vi "WRO_Main.vi"() -> ()   [LabVIEW 2014]
uses:
  <vilib>/myRIO/Instrument Drivers/Onboard IO/DIO/typedefs/DIO Reference.ctl
  <vilib>/myRIO/Common/Instrument Driver Framework/Utilities/typedefs/myRIO Generic Hardware Reference.ctl
  <vilib>/myRIO/Common/Instrument Driver Framework/Utilities/typedefs/Hardware Version Enum.ctl
  <vilib>/myRIO/Common/Instrument Driver Framework/Utilities/typedefs/myRIO v1.0 Reference.ctl
  <vilib>/myRIO/Common/Instrument Driver Framework/Utilities/typedefs/Generic FPGA Reference.ctl
  <vilib>/myRIO/Common/Instrument Driver Framework/myRIO v1.0/DIO/typedefs/DIO Channels List.ctl
  <vilib>/myRIO/Common/Instrument Driver Framework/myRIO v1.0/DIO/typedefs/DIO Channels Enum.ctl
  <vilib>/userdefined/High Color/nirio_resource_hc.ctl
  <vilib>/myRIO/Common/Instrument Driver Framework/Utilities/vis/Is FPGA Ref Available.vi
  <vilib>/myRIO/Common/Instrument Driver Framework/myRIO v1.0/DIO/vis/myRIO v1.1 Open DIO.vi
  <vilib>/myRIO/Instrument Drivers/Onboard IO/DIO/vis/Write.vi
  <vilib>/myRIO/Instrument Drivers/Onboard IO/DIO/vis/Read.vi
  <vilib>/myRIO/Common/Instrument Driver Framework/Utilities/vis/Validate Channels.vi
  <vilib>/myRIO/Common/Instrument Driver Framework/myRIO v1.0/DIO/vis/myRIO v1.0 Reserve DIO.vi
  <vilib>/myRIO/Common/Instrument Driver Framework/myRIO v1.0/Resource Manager/vis/myRIO v1.0 Reserve Channel List.vi
  <vilib>/myRIO/Common/Instrument Driver Framework/myRIO v1.0/DIO/vis/myRIO v1.0 Build MUX Configuration DIO.vi
  <vilib>/myRIO/Common/Instrument Driver Framework/myRIO v1.0/Resource Manager/vis/myRIO v1.0 Reserve Channel.vi
  <vilib>/myRIO/Common/Instrument Driver Framework/myRIO v1.0/Resource Manager/vis/myRIO v1.0 Unreserve Channel.vi
  <vilib>/myRIO/Common/Instrument Driver Framework/myRIO v1.0/Resource Manager/vis/myRIO v1.0 Create Configuration List.vi
  <vilib>/myRIO/Common/Instrument Driver Framework/myRIO v1.0/Resource Manager/vis/myRIO v1.0 Build Mutex Name.vi
  <vilib>/Utility/VariantDataType/GetNumericInfo.vi
  <vilib>/Utility/error.llb/Error Cluster From Error Code.vi
  <vilib>/myRIO/Common/Instrument Driver Framework/myRIO v1.0/myRIO v1.1 Open.vi
  <vilib>/myRIO/Common/Instrument Driver Framework/Utilities/vis/IO Manager.vi
  <vilib>/myRIO/Common/Instrument Driver Framework/Utilities/vis/Configuration Manager.vi
  <vilib>/myRIO/Common/Instrument Driver Framework/myRIO v1.0/Resource Manager/vis/myRIO v1.0 Configure IO.vi
  <vilib>/myRIO/Common/Instrument Driver Framework/myRIO v1.0/myRIO v1.0 Close.vi
  <vilib>/myRIO/Common/Instrument Driver Framework/myRIO v1.0/DIO/vis/myRIO v1.0 Write DIO.vi
  <vilib>/myRIO/Common/Instrument Driver Framework/myRIO v1.0/DIO/vis/myRIO v1.0 Read DIO.vi
  <vilib>/myRIO/Express VI/Onboard Devices/LED/LED Express VI.xnode
  <vilib>/myRIO/Instrument Drivers/Onboard IO/DIO/vis/myRIO DIO Open.xnode
  <vilib>/myRIO/Express VI/Onboard Devices/Button/Button Express VI.xnode
  <vilib>/myRIO/Instrument Drivers/Onboard IO/DIO/DIO.lvlib
panel:
  in  "2: 굴릴각도":dbl=60.0
  in  "2: 공각도":dbl=230.0
  in  "흰/검 반 값":dbl=0.3
  in  "흰색과 밖 차이값":dbl=0.15
  in  "6: 왼쪽각도":dbl=245.0
  in  "6: 앞쪽각도":dbl=125.0
  in  "5: 앞쪽각도":dbl=245.0
  in  "4: 뒷쪽각도":dbl
  in  "5: 오른각도":dbl=120.0
  in  "4: 오른각도":dbl=122.0
  in  "정지할 차이값":dbl=0.08
  # "조정해야하는 프로젝트\n:    Main ,  ball , BBO(색상값) , 스페어, Max"
  # "마지막꺼 초조절"
  # "로봇 수평맞추거나 움직이는 부분"
  # "서브모터 각도"
  # "60"
  # "230"
  # "2번 바꿨을 경우엔  Goo0FF확인- 중간값"
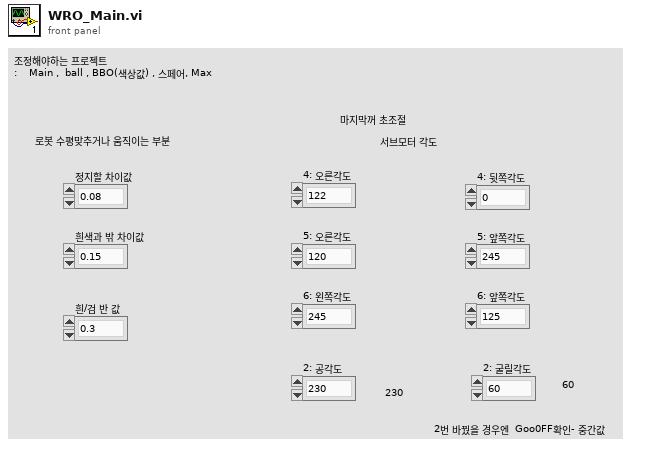
[diagram p1: front panel]
types:
  T1 = typedef "DIO.lvlib/DIO Reference.ctl" = cluster{"myRIO Reference":T2, "DIO Channels List":T6}
  T2 = typedef "myRIO Generic Hardware Reference.ctl" = cluster{"myRIO Model":T3, "myRIO Hardware Reference":T4}
  T3 = typedef "Hardware Version Enum.ctl" = enum16{"Unknown", "myRIO-1900", "myRIO-1950"}
  T4 = typedef "myRIO v1.0 Reference.ctl" = cluster{"Generic FPGA Reference":T5, "Allow multiple opens":bool}
  T5 = typedef "Generic FPGA Reference.ctl" = refnum<k20>
  T6 = typedef "DIO Channels List.ctl" = T7[]
  T7 = typedef "DIO Channels Enum.ctl" = enum16{"Not Connected", "C/DIO0", "C/DIO1", "C/DIO2", "C/DIO3", "C/DIO4", "C/DIO5", "C/DIO6", "C/DIO7", "A/DIO0", "A/DIO1", "A/DIO2", "A/DIO3", "A/DIO4", "A/DIO5", "A/DIO6", "A/DIO7", "A/DIO8", "A/DIO9", "A/DIO10", "A/DIO11", "A/DIO12", "A/DIO13", "A/DIO14", "A/DIO15", "B/DIO0", "B/DIO1", "B/DIO2", "B/DIO3", "B/DIO4", "B/DIO5", "B/DIO6", "B/DIO7", "B/DIO8", "B/DIO9", "B/DIO10", "B/DIO11", "B/DIO12", "B/DIO13", "B/DIO14", "B/DIO15", "LED0", "LED1", "LED2", "LED3", "Button0"}
  T8 = typedef "nirio_resource_hc.ctl" = tag
  T9 = cluster{"정지할 차이값":dbl, "흰색과 밖 차이값":dbl, "흰/검 반 값 ":dbl}
  T10 = cluster{"4: 오른각도":dbl, "4: 뒷쪽각도":dbl, "5: 오른각도":dbl, "5: 앞쪽각도":dbl, "6: 왼쪽각도":dbl, "6: 앞쪽각도":dbl}
  T11 = cluster{cluster{"정지할 차이값":dbl, "흰색과 밖 차이값":dbl, "흰/검 반 값 ":dbl}, cluster{"4: 오른각도":dbl, "4: 뒷쪽각도":dbl, "5: 오른각도":dbl, "5: 앞쪽각도":dbl, "6: 왼쪽각도":dbl, "6: 앞쪽각도":dbl}, cluster{"2: 공각도":dbl, "2: 굴릴각도":dbl}}
  T12 = cluster{"Global Rectangle":i32[], "Contours":cluster{"Contour Type":u32, "ROI Type":u32, "Points":i32[]}[]}
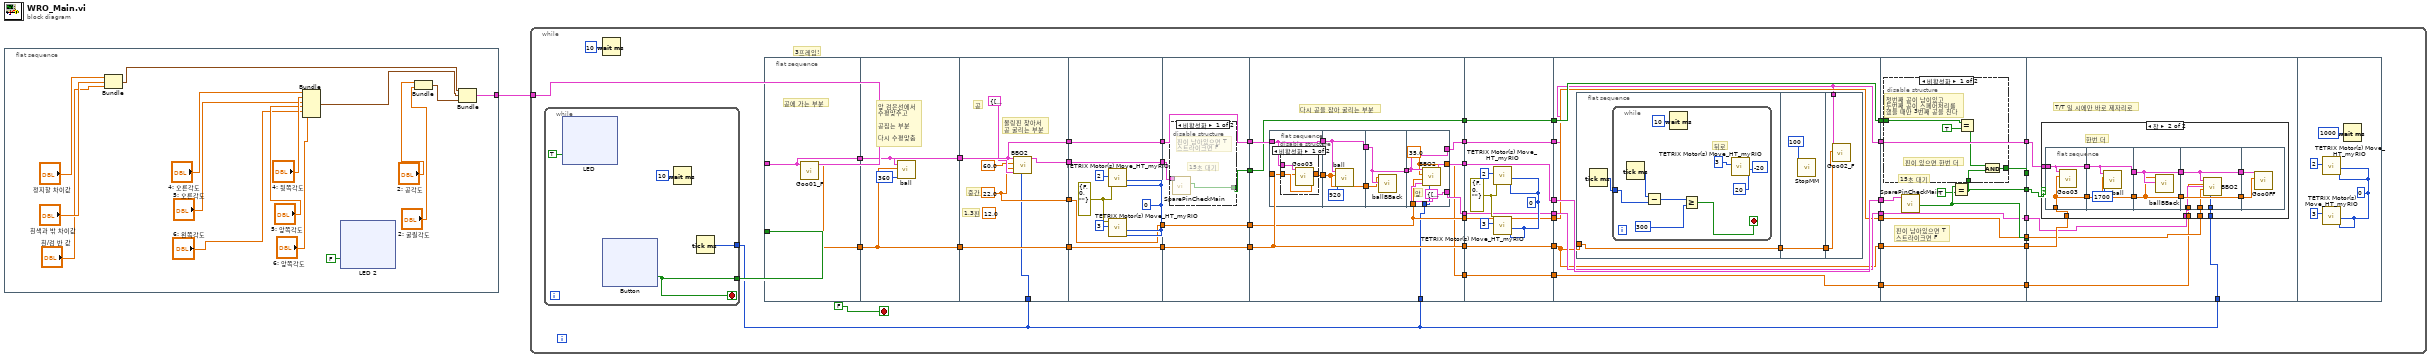
[diagram p0: block diagram]
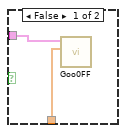
[diagram p5: hidden frame]
diagram:
  n1 = flat-sequence {
    tunnel: [w3] -> w1
    frame #0 {
      n2 = Bundle("정지할 차이값"="정지할 차이값", "흰색과 밖 차이값"="흰색과 밖 차이값", "흰/검 반 값"="흰/검 반 값") -> (w6:T9)  [unwired: 1 in]
      n3 = Bundle("4: 오른각도"="4: 오른각도", "4: 뒷쪽각도"="4: 뒷쪽각도", "5: 오른각도"="5: 오른각도", "5: 앞쪽각도"="5: 앞쪽각도", "6: 왼쪽각도"="6: 왼쪽각도", "6: 앞쪽각도"="6: 앞쪽각도") -> (w5:T10)  [unwired: 1 in]
      n4 = xnode "LED 2"("LED0"=FALSE) -> ()  [unwired: 1 in, 1 out]
      n5 = Bundle("2: 공각도"="2: 공각도", "2: 굴릴각도"="2: 굴릴각도") -> (w4:cluster{"2: 공각도":dbl, "2: 굴릴각도":dbl})  [unwired: 1 in]
      n6 = Bundle(w6, w5, w4) -> (w3:T11)  [unwired: 1 in]
    }
  }
  n7 = while {
    tunnel: w1 -> [w101]
    stop <- FALSE stop-if-true
    # "3프레임!"
    n8 = while {
      tunnel: [w104] -> w79
      tunnel: [w103] -> w53
      stop <- w104 stop-if-true
      n9 = xnode "LED"("LED0"=TRUE) -> ()  [unwired: 1 in, 1 out]
      n10 = xnode "Button"() -> ("Value"=w104:bool)  [unwired: 1 in, 1 out]
      n11 = Wait (ms)(milliseconds to wait=u32 10 ("대기 시간(ms)")) -> ()  [unwired: 1 out]
      n12 = Tick Count (ms)() -> (millisecond timer value=w103:u32)
    }
    n13 = Wait (ms)(milliseconds to wait=u32 10 ("대기 시간(ms)")) -> ()  [unwired: 1 out]
    n14 = flat-sequence {
      tunnel: [w178] -> w100
      tunnel: [w177] -> w99
      tunnel: w101 -> [w178]
      tunnel: w79 -> [_]
      tunnel: w100 -> [w181]
      tunnel: [w181] -> w98
      tunnel: [w180] -> w97
      tunnel: w99 -> [w180]
      tunnel: w98 -> [w187]
      tunnel: [w188] -> w96
      tunnel: [w187] -> w95
      tunnel: [w186] -> w94
      tunnel: w97 -> [w186]
      tunnel: [w184] -> w74
      tunnel: w53 -> [w182]
      tunnel: [w192] -> w93
      tunnel: w96 -> [w192]
      tunnel: [w191] -> w92
      tunnel: w95 -> [w191]
      tunnel: [w190] -> w91
      tunnel: w94 -> [w190]
      tunnel: w74 -> [w189]
      tunnel: [w189] -> w73
      tunnel: [w201] -> w90
      tunnel: w93 -> [w200]
      tunnel: [w199] -> w89
      tunnel: w92 -> [w199]
      tunnel: w91 -> [w198]
      tunnel: [w198] -> w88
      tunnel: w73 -> [w197]
      tunnel: [w197] -> w72
      tunnel: w90 -> [w211]
      tunnel: [w211] -> w87
      tunnel: w89 -> [w217]
      tunnel: [w215] -> w86
      tunnel: [w214] -> w85
      tunnel: w88 -> [w213]
      tunnel: [w213] -> w84
      tunnel: [w207] -> w75
      tunnel: w72 -> [w206]
      tunnel: [w206] -> w70
      tunnel: [w205] -> w54
      tunnel: w53 -> [w204]
      tunnel: [w241] -> w69
      tunnel: w87 -> [w241]
      tunnel: [w239] -> w67
      tunnel: w86 -> [w239]
      tunnel: [w238] -> w65
      tunnel: w85 -> [w238]
      tunnel: w84 -> [w237]
      tunnel: [w237] -> w63
      tunnel: [w236] -> w61
      tunnel: w75 -> [w236]
      tunnel: [w235] -> w59
      tunnel: w70 -> [w235]
      tunnel: [w234] -> w55
      tunnel: w54 -> [w234]
      tunnel: w69 -> [w253]
      tunnel: [w253] -> w68
      tunnel: w67 -> [w252]
      tunnel: [w252] -> w66
      tunnel: w65 -> [w246]
      tunnel: [w246] -> w64
      tunnel: w63 -> [w247]
      tunnel: [w247] -> w62
      tunnel: w61 -> [w251]
      tunnel: [w251] -> w60
      tunnel: w59 -> [w250]
      tunnel: [w250] -> w58
      tunnel: [w245] -> w57
      tunnel: w55 -> [w245]
      tunnel: [w278] -> w83
      tunnel: w68 -> [w279]
      tunnel: w66 -> [w277]
      tunnel: [w272] -> w82
      tunnel: w64 -> [w272]
      tunnel: w62 -> [w276]
      tunnel: [w276] -> w81
      tunnel: [w275] -> w78
      tunnel: [w273] -> w77
      tunnel: [w271] -> w76
      tunnel: w60 -> [w271]
      tunnel: [w270] -> w71
      tunnel: w58 -> [w270]
      tunnel: w57 -> [w269]
      tunnel: [w269] -> w56
      tunnel: w83 -> [_]
      tunnel: w82 -> [w291]
      tunnel: w81 -> [w290]
      tunnel: w78 -> [_]
      tunnel: w77 -> [w289]
      tunnel: w76 -> [w288]
      tunnel: w71 -> [w287]
      tunnel: w56 -> [w286]
      tunnel: w53 -> [w285]
      frame #0 {
        # "공에 가는 부분"
        n15 = call "Goo01_F.vi"("클러스터"=w178) -> ("ColorSensor"=w177:dbl[])  [unwired: 10 in]
      }
      frame #1 {
        # "앞 검은선에서 \n수평맞추고\n\n공집는 부분\n\n다시 수평맞춤"
        n16 = call "ball.vi"("공한테 가는(뒤로) 초"=u32 360, "ColorSensor"=w180, "클러스터"=w181) -> ()  [unwired: 9 in]
      }
      frame #2 {
        (unwired) 12.0 ("카메라 X")
        w184 = 22.0 ("카메라 X")
        # "1,3핀"
        # "중간"
        # "공"
        # "볼링핀 찾아서\n공 굴리는 부분"
        n17 = call "BBO2.vi"("시작시간 값"=w182, "ROI 2"=T12 {"Global Rectangle"=[499, 445, 758, 571], "Contours"=[{"Contour Type"=0, "ROI Type"=3, "Points"=[499, 445, 758, 571]}]} ("ROI"), "카메라 X"=w184, "핀간격"=60.0, "클러스터"=w187) -> ("ROI"=w188:T12)  [unwired: 6 in]
      }
      frame #3 {
        w193 = errorcluster {"status"=FALSE, "code"=0, "source"=""} ("error in (no error)")
        w194 = 0
        n18 = call <vilib>:"TETRIX Motor(s) Move_HT_myRIO.vi"("Motor 2 Power (-100 to 100)\n0 = Stop/Brake\n-128 = Stop/Coast"=w194, "Motor 1 Power (-100 to 100)\n0 = Stop/Brake\n-128 = Stop/Coast"=w194, "Controller Daisy Chain Position: 1 - 4"=u8 2, "error in (no error)"=w193) -> ()  [unwired: 5 in, 1 out]
        n19 = call <vilib>:"TETRIX Motor(s) Move_HT_myRIO.vi"("Motor 2 Power (-100 to 100)\n0 = Stop/Brake\n-128 = Stop/Coast"=w194, "Motor 1 Power (-100 to 100)\n0 = Stop/Brake\n-128 = Stop/Coast"=w194, "Controller Daisy Chain Position: 1 - 4"=u8 3, "error in (no error)"=w193) -> ()  [unwired: 5 in, 1 out]
      }
      frame #4 {
        n20 = disable-structure shown="비활성화" {
          disable-tunnel: [w203 _] -> w201
          disable-tunnel: w200 -> [w202 _]
          frame Disabled {
            # "15초 대기"
            # "핀이 남아있으면 T\n스트라이크면 F"
            n21 = call "SparePinCheckMain.vi"("ROI"=w202) -> ("불리언"=w203:bool)  [unwired: 10 in]
          }
          frame Enabled {
          }
        }
      }
      frame #5 {
        # "다시 공을 잡아 굴리는 부분"
        n22 = flat-sequence {
          tunnel: w217 -> [w219]
          tunnel: [w219] -> w216
          tunnel: w213 -> [w218]
          tunnel: [w218] -> w212
          tunnel: w216 -> [w225]
          tunnel: [w225] -> w210
          tunnel: w212 -> [w223]
          tunnel: [w223] -> w208
          tunnel: w210 -> [w227]
          tunnel: [w227] -> w209
          tunnel: w208 -> [w226]
          tunnel: w209 -> [w232]
          tunnel: [w233] -> w215
          tunnel: [w232] -> w214
          tunnel: [w231] -> w207
          tunnel: w206 -> [w230]
          tunnel: [w229] -> w205
          tunnel: w204 -> [w228]
          frame #0 {
            n23 = disable-structure shown="비활성화" {
              disable-tunnel: w219 -> [w221 _]
              disable-tunnel: w218 -> [w220 w222]
              disable-tunnel: [_ w222] -> _
              frame Disabled {
                n24 = call "Goo03.vi"("ColorSensor"=w220, "클러스터"=w221) -> ()  [unwired: 10 in]
              }
              frame Enabled {
              }
            }
          }
          frame #1 {
            n25 = call "ball.vi"("공한테 가는(뒤로) 초"=u32 920, "ColorSensor"=w223, "클러스터"=w225) -> ()  [unwired: 9 in]
          }
          frame #2 {
            n26 = call "ballBBack.vi"("클러스터"=w227, "ColorSensor"=w226) -> ()  [unwired: 10 in]
          }
          frame #3 {
            w229 = 35.0 ("핀간격")
            w231 = T12 {"Global Rectangle"=[536, 448, 795, 574], "Contours"=[{"Contour Type"=0, "ROI Type"=3, "Points"=[536, 448, 795, 574]}]} ("ROI")
            # "앞"
            n27 = call "BBO2.vi"("시작시간 값"=w228, "ROI 2"=w231, "카메라 X"=w230, "핀간격"=w229, "클러스터"=w232) -> ("ROI"=w233:T12)  [unwired: 6 in]
          }
        }
      }
      frame #6 {
        w240 = errorcluster {"status"=FALSE, "code"=0, "source"=""} ("error in (no error)")
        w244 = 0
        n28 = call <vilib>:"TETRIX Motor(s) Move_HT_myRIO.vi"("Motor 2 Power (-100 to 100)\n0 = Stop/Brake\n-128 = Stop/Coast"=w244, "Motor 1 Power (-100 to 100)\n0 = Stop/Brake\n-128 = Stop/Coast"=w244, "Controller Daisy Chain Position: 1 - 4"=u8 2, "error in (no error)"=w240) -> ()  [unwired: 5 in, 1 out]
        n29 = call <vilib>:"TETRIX Motor(s) Move_HT_myRIO.vi"("Motor 2 Power (-100 to 100)\n0 = Stop/Brake\n-128 = Stop/Coast"=w244, "Motor 1 Power (-100 to 100)\n0 = Stop/Brake\n-128 = Stop/Coast"=w244, "Controller Daisy Chain Position: 1 - 4"=u8 3, "error in (no error)"=w240) -> ()  [unwired: 5 in, 1 out]
      }
      frame #7 {
        n30 = flat-sequence {
          tunnel: [w254] -> w248
          tunnel: w247 -> [w254]
          tunnel: [w265] -> w249
          tunnel: w248 -> [w265]
          tunnel: w249 -> [w268]
          tunnel: w246 -> [w267]
          frame #0 {
            n31 = Tick Count (ms)() -> (millisecond timer value=w255:u32)
            n32 = while {
              tunnel: w255 -> [w260]
              stop <- w258 stop-if-true
              # "뒤로"
              n33 = Tick Count (ms)() -> (millisecond timer value=w261:u32)
              n34 = Subtract(x=w261, y=w260) -> (x-y=w259:u32)
              n35 = Wait (ms)(milliseconds to wait=u32 10 ("대기 시간(ms)")) -> ()  [unwired: 1 out]
              n36 = Greater Or Equal?(x=w259, y=u32 300) -> (x >= y?=w258:bool)
              n37 = call <vilib>:"TETRIX Motor(s) Move_HT_myRIO.vi"("Motor 2 Power (-100 to 100)\n0 = Stop/Brake\n-128 = Stop/Coast"=i8 20 ("Motor 2 Power (-100 to 100)\n0 = Stop/Brake\n-128 = Stop/Coast"), "Motor 1 Power (-100 to 100)\n0 = Stop/Brake\n-128 = Stop/Coast"=i8 -20 ("Motor 1 Power (-100 to 100)\n0 = Stop/Brake\n-128 = Stop/Coast"), "Controller Daisy Chain Position: 1 - 4"=u8 3) -> ()  [unwired: 6 in, 1 out]
            }
          }
          frame #1 {
            n38 = call "StopMM.vi"("대기 시간(ms)"=u32 100) -> ()  [unwired: 11 in]
          }
          frame #2 {
            n39 = call "Goo02_F.vi"("ColorSensor 2"=w268, "클러스터"=w267) -> ()  [unwired: 10 in]
          }
        }
      }
      frame #8 {
        # "핀이 남아있으면 T\n스트라이크면 F"
        n40 = call "SparePinCheckMain.vi"("ROI"=w277) -> ("불리언"=w275:bool)  [unwired: 10 in]
        n41 = Equal?(x=w275, y=TRUE) -> (x = y?=w273:bool)
        n42 = disable-structure shown="비활성화" {
          disable-tunnel: w279 -> [w284 _]
          disable-tunnel: [w283 _] -> w278
          disable-tunnel: w273 -> [w280 _]
          frame Disabled {
            # "핀이 있으면 한번 더"
            # "15초 대기"
            # "첫번째 공이 남이있고\n두번째 공이 스페어처리를\n했을 때만 3번째 공을 친다"
            n43 = Equal?(x=w284, y=TRUE) -> (x = y?=w281:bool)
            n44 = And(x=w281, y=w280) -> (x .and. y?=w283:bool)
          }
          frame Enabled {
          }
        }
      }
      frame #9 {
        # "T/T 일 시에만 바로 제자리로"
        n45 = case shown="참" w289 {
          tunnel: w291 -> [w293 w307]
          tunnel: w290 -> [w292 w304]
          tunnel: w288 -> [_ w297]
          tunnel: w287 -> [_ w296]
          tunnel: w286 -> [_ w295]
          tunnel: w285 -> [_ w294]
          frame False {
            n46 = call "Goo0FF.vi"("ColorSensor"=w292, "클러스터"=w293) -> ()  [unwired: 10 in]
          }
          frame True {
            # "한번 더"
            n47 = flat-sequence {
              tunnel: w307 -> [w309]
              tunnel: [w309] -> w306
              tunnel: w304 -> [w308]
              tunnel: [w308] -> w303
              tunnel: w306 -> [w312]
              tunnel: [w312] -> w301
              tunnel: w303 -> [w311]
              tunnel: [w311] -> w299
              tunnel: w301 -> [w314]
              tunnel: [w314] -> w300
              tunnel: w299 -> [w313]
              tunnel: [w313] -> w298
              tunnel: w300 -> [w320]
              tunnel: [w320] -> w305
              tunnel: w298 -> [w319]
              tunnel: [w319] -> w302
              tunnel: w297 -> [w318]
              tunnel: w296 -> [w317]
              tunnel: w295 -> [w316]
              tunnel: w294 -> [w315]
              tunnel: w305 -> [w322]
              tunnel: w302 -> [w321]
              frame #0 {
                n48 = call "Goo03.vi"("ColorSensor"=w308, "클러스터"=w309) -> ()  [unwired: 10 in]
              }
              frame #1 {
                n49 = call "ball.vi"("공한테 가는(뒤로) 초"=u32 1700, "ColorSensor"=w311, "클러스터"=w312) -> ()  [unwired: 9 in]
              }
              frame #2 {
                n50 = call "ballBBack.vi"("클러스터"=w314, "ColorSensor"=w313) -> ()  [unwired: 10 in]
              }
              frame #3 {
                n51 = call "BBO2.vi"("시작시간 값"=w315, "ROI 2"=w318, "카메라 X"=w317, "핀간격"=w316, "클러스터"=w320) -> ()  [unwired: 6 in, 1 out]
              }
              frame #4 {
                n52 = call "Goo0FF.vi"("ColorSensor"=w321, "클러스터"=w322) -> ()  [unwired: 10 in]
              }
            }
          }
        }
      }
      frame #10 {
        w326 = 0
        n53 = call <vilib>:"TETRIX Motor(s) Move_HT_myRIO.vi"("Motor 2 Power (-100 to 100)\n0 = Stop/Brake\n-128 = Stop/Coast"=w326, "Motor 1 Power (-100 to 100)\n0 = Stop/Brake\n-128 = Stop/Coast"=w326, "Controller Daisy Chain Position: 1 - 4"=u8 2) -> ()  [unwired: 6 in, 1 out]
        n54 = call <vilib>:"TETRIX Motor(s) Move_HT_myRIO.vi"("Motor 2 Power (-100 to 100)\n0 = Stop/Brake\n-128 = Stop/Coast"=w326, "Motor 1 Power (-100 to 100)\n0 = Stop/Brake\n-128 = Stop/Coast"=w326, "Controller Daisy Chain Position: 1 - 4"=u8 3) -> ()  [unwired: 6 in, 1 out]
        n55 = Wait (ms)(milliseconds to wait=u32 1000 ("대기 시간(ms)")) -> ()  [unwired: 1 out]
      }
    }
  }
